vi "cross_product.vi"(9 "Vect 2":cluster{"X":sgl, "Y":sgl, "Z":sgl}, 10 "Vect 1":cluster{"X":sgl, "Y":sgl, "Z":sgl}) -> (2 "Vect Out":cluster{"X":sgl, "Y":sgl, "Z":sgl})   [LabVIEW 2020]
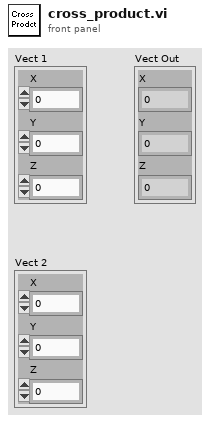
[diagram p1: front panel]
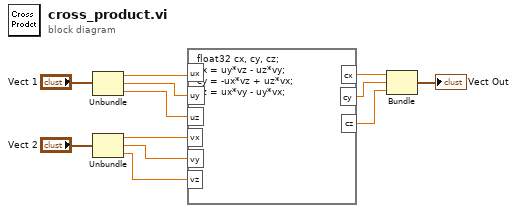
[diagram p0: block diagram]
diagram:
  n1 = Unbundle("Vect 1") -> ("X"=w10:sgl, "Y"=w9:sgl, "Z"=w8:sgl)
  n2 = Unbundle("Vect 2") -> ("X"=w7:sgl, "Y"=w6:sgl, "Z"=w5:sgl)
  n3 = formula code="float32 cx, cy, cz;\ncx = uy*vz - uz*vy;\ncy = -ux*vz + uz*vx;\ncz = ux*vy - uy*vx;"("ux"=w10, "uy"=w9, "uz"=w8, "vx"=w7, "vy"=w6, "vz"=w5) -> ("cx"=w4:sgl, "cy"=w3:sgl, "cz"=w2:sgl)
  n4 = Bundle(w4, w3, w2) -> (→"Vect Out":cluster{sgl, sgl, sgl})  [unwired: 1 out]
